vi "自定义ADC.vi"(8 "Vref V":dbl=2.56, 11 "输入 V":dbl) -> (2 "数字编码":dbl[](array[numeric]))   [LabVIEW 2020]
uses:
  <vilib>/express/express arith-compare/Formula/XNode/ExpressFormulaBlockNode.xnode
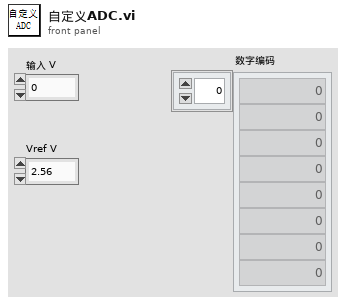
[diagram p1: front panel]
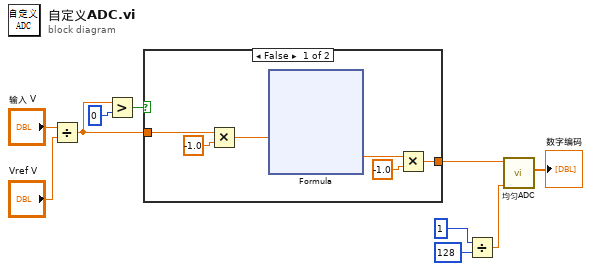
[diagram p0: block diagram]
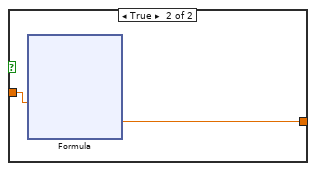
[diagram p2: hidden frame]
diagram:
  n1 = Divide(x="输入 V", y="Vref V") -> (x/y=w1:dbl)
  n2 = Greater?(x=w1, y=0) -> (0:w3:bool)
  n3 = case shown="False" w3 {
    tunnel: [w11 w26] -> w2
    tunnel: w1 -> [w15 w25]
    frame False {
      n4 = Multiply(x=w15, y=-1.0) -> (x*y=w14:dbl)
      n5 = xnode "Formula"("X"=w14) -> ("Result"=w12:dbl)  [unwired: 1 in, 1 out]
      n6 = Multiply(x=w12, y=-1.0) -> (x*y=w11:dbl)
    }
    frame True {
      n7 = xnode "Formula"("X"=w25) -> ("Result"=w26:dbl)  [unwired: 1 in, 1 out]
    }
  }
  n8 = Divide(x=1, y=128) -> (x/y=w5:dbl)
  n9 = call "均匀ADC.vi"("量化阶 V"=w5, "输入的模拟信号取样值 V"=w2) -> ("数字编码"=→"数字编码":dbl[])  [unwired: 9 in]
